vi "BK Precision 8500B Series Run Constant Current Transient.vi"() -> ()   [LabVIEW 2024]
doc: "Exemplifies how to configure and run a Constant Current transient operation in which the load will continuously toggle between level A and level B value with the specified time. It also monitors the current during this test."
uses:
  BK Precision 8500B Series.lvlib
panel:
  in  "B Width (1s)":dbl=1.0 min=0.0 max=3600.0 step=1.0 format="%#.6f"
  in  "B Level Value (2.000)":dbl=2.0 min=0.0 max=240.0 step=1.0 format="%.3f"
  in  "A Width (1s)":dbl=1.0 min=0.0 max=3600.0 step=1.0 format="%#.6f"
  in  "A Level Value (1.000)":dbl=1.0 min=0.0 max=240.0 step=1.0 format="%.3f"
  out "Current":dbl format="%_6g"
  out "Voltage":dbl format="%_6f"
  in  "Transient Mode (0:Continuous)":u16(ring) items=["Continuous", "Pulse", "Toggle"]
  in  "?":bool
  in  "VISA resource name":refnum<visa-resource-name>
  in  "Serial Configuration":cluster{"Baud Rate":u32}={"Baud Rate"=9600} {"Baud Rate" items=["300"=300, "600"=600, "1200"=1200, "2400"=2400, "4800"=4800, "9600"=9600, "19200"=19200]}
  # "(c) 2019 B&K Precision Corporation.  ALL RIGHTS RESERVED."
  # "s"
  # "s"
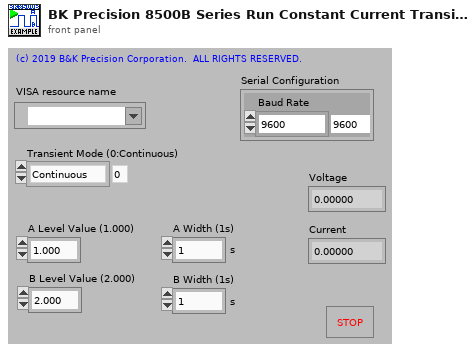
[diagram p1: front panel]
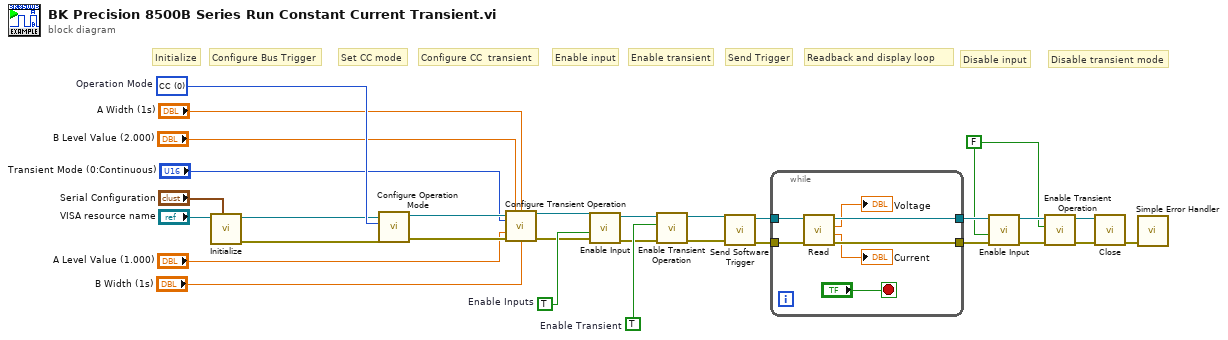
[diagram p0: block diagram]
diagram:
  w16 = u16 0 items=["CC", "CV", "CR", "CW"]  # Operation Mode
  w17 = FALSE
  w24 = TRUE  # Enable Inputs
  w28 = TRUE  # Enable Transient
  # "Readback and display loop"
  # "Disable transient mode"
  # "Disable input"
  # "Send Trigger"
  # "Enable input"
  # "Enable transient"
  # "Configure CC  transient"
  # "Set CC mode"
  # "Configure Bus Trigger"
  # "Initialize"
  n1 = call "Initialize.vi"("Serial Configuration"="Serial Configuration", "VISA resource name"="VISA resource name") -> ("error out"=w14:errorcluster, "VISA resource name out"=w15:refnum<visa-resource-name>)  [unwired: 8 in]
  n2 = call "Configure Operation Mode.vi"("error in (no error)"=w14, "Operation Mode (0:CC)"=w16, "VISA resource name"=w15) -> ("error out"=w11:errorcluster, "VISA resource name out"=w13:refnum<visa-resource-name>)  [unwired: 7 in]
  n3 = call "Configure Transient Operation.vi"("VISA resource name"=w13, "B Level Value (2.000)"="B Level Value (2.000)", "A Width (1s)"="A Width (1s)", "Transient Mode (0:Continuous)"="Transient Mode (0:Continuous)", "A Level Value (1.000)"="A Level Value (1.000)", "error in (no error)"=w11, "B Width (1s)"="B Width (1s)") -> ("VISA resource name out"=w9:refnum<visa-resource-name>, "error out"=w10:errorcluster)  [unwired: 7 in]
  n4 = call "Enable Input.vi"("error in (no error)"=w10, "Enable Input (F: False)"=w24, "VISA resource name"=w9) -> ("error out"=w7:errorcluster, "VISA resource name out"=w8:refnum<visa-resource-name>)  [unwired: 7 in]
  n5 = call "Enable Transient Operation.vi"("error in (no error)"=w7, "Enable Transient (T: Enable)"=w28, "VISA resource name"=w8) -> ("error out"=w5:errorcluster, "VISA resource name out"=w6:refnum<visa-resource-name>)  [unwired: 7 in]
  n6 = call "Send Software Trigger.vi"("error in (no error)"=w5, "VISA resource name"=w6) -> ("error out"=w26:errorcluster, "VISA resource name out"=w27:refnum<visa-resource-name>)  [unwired: 8 in]
  n7 = while {
    tunnel: [w34] -> w23
    tunnel: w27 -> [w35]
    tunnel: [w33] -> w22
    tunnel: w26 -> [w36]
    stop <- "?" stop-if-true
    n8 = call "Read.vi"("error in (no error)"=w36, "VISA resource name"=w35) -> ("error out"=w33:errorcluster, "Current"=→"Current":dbl, "Voltage"=→"Voltage":dbl, "VISA resource name out"=w34:refnum<visa-resource-name>)  [unwired: 6 in]
  }
  n9 = call "Enable Input.vi"("error in (no error)"=w22, "Enable Input (F: False)"=w17, "VISA resource name"=w23) -> ("error out"=w21:errorcluster, "VISA resource name out"=w20:refnum<visa-resource-name>)  [unwired: 7 in]
  n10 = call "Enable Transient Operation.vi"("error in (no error)"=w21, "Enable Transient (T: Enable)"=w17, "VISA resource name"=w20) -> ("error out"=w18:errorcluster, "VISA resource name out"=w19:refnum<visa-resource-name>)  [unwired: 7 in]
  n11 = call "Close.vi"("error in (no error)"=w18, "VISA resource name"=w19) -> ("error out"=w25:errorcluster)  [unwired: 9 in]
  n12 = call <vilib>:"Simple Error Handler.vi"("error in (no error)"=w25) -> ()  [unwired: 4 in, 5 out]
